vi "Go.vi"(8 "Timing Data (Go Down and Dispense)":T1(array[cluster]), 9 "Timing Data":dbl[](array[numeric]), 10 "Control In":T2={"I-O.lvclass"=refnum, "Motion.lvclass"=refnum, "Dispenser.lvclass"=refnum}, 11 "C4 Dispense in":refnum<class "Iterative Dispense.lvclass">) -> (2 "Control Out":T2, 3 "C4 Dispense Out":refnum<class "Iterative Dispense.lvclass">)   [LabVIEW 2016, in "Iterative Dispense.lvclass"]
uses:
  Iterative Dispense.lvclass
  Controller/Controllers.ctl
  Controller/I-O/I-O.lvclass
  Controller/Motion/A3200/A3200.lvclass
  Controller/Dispenser/Dispenser.lvclass
  Controller/Motion/Motion.lvclass
  Iterative Dispense.lvclass/Iterative Dispense.ctl
  Controller/Controller.lvclass
panel:
  out "deleted portion":dbl[][](array[numeric])
  out "array w/ subset deleted":dbl[][][](array[numeric])
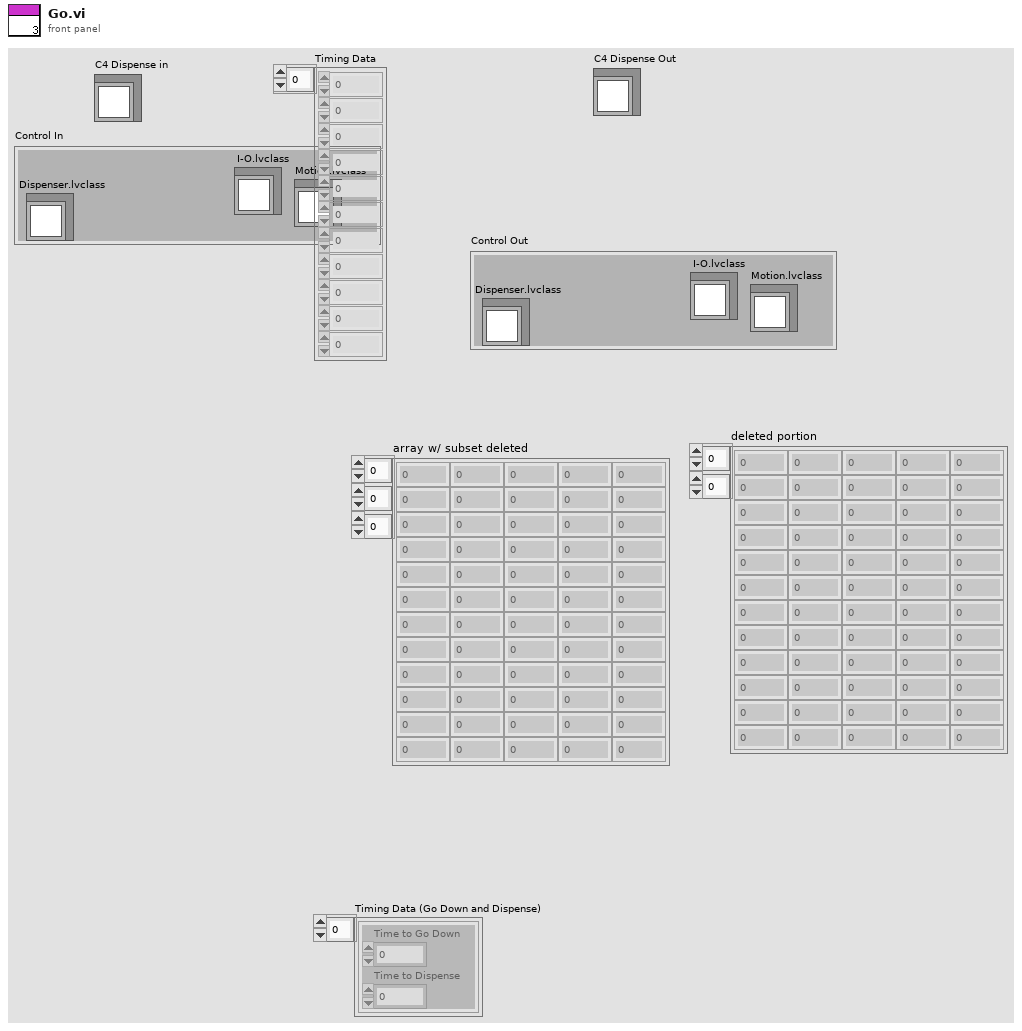
[diagram p1: front panel]
types:
  T1 = cluster{"Time to Go Down":dbl, "Time to Dispense":dbl}[]
  T2 = typedef "Controller.lvclass/Controllers.ctl" = cluster{"I-O.lvclass":refnum<class "I-O.lvclass">, "Motion.lvclass":refnum<class "Motion.lvclass">, "Dispenser.lvclass":refnum<class "Dispenser.lvclass">}
  T3 = typedef "Iterative Dispense.lvclass/Glue Step Enum.ctl" = enum16{"Baseplate to Kapton", "Kapton to Sensor"}
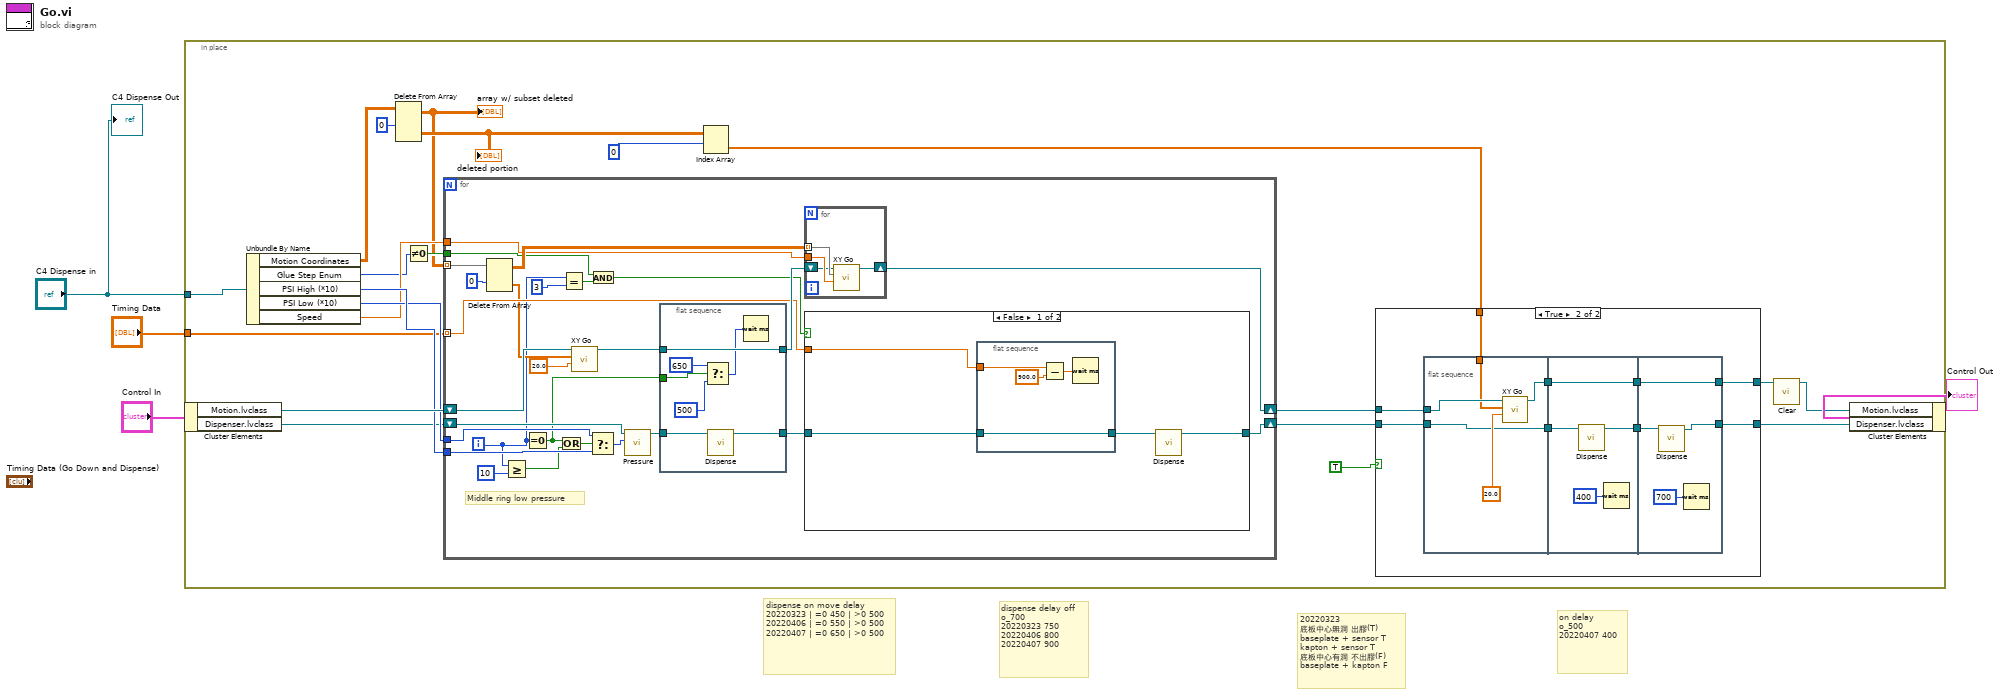
[diagram p0: block diagram]
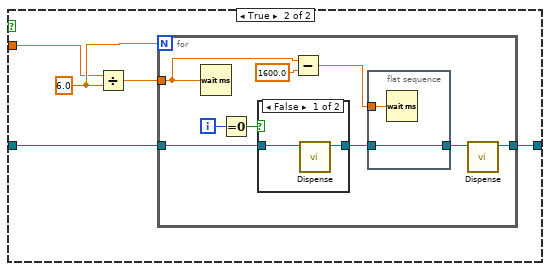
[diagram p3: hidden frame]
diagram:
  # "20220323\n底板中心無洞 出膠(T)\nbaseplate + sensor T\nkapton + sensor T\n底板中心有洞 不出膠(F)\nbaseplate + kapton F"
  # "on delay\no_500\n20220407 400"
  # "dispense delay off\no_700\n20220323 750\n20220406 800\n20220407 900"
  # "dispense on move delay\n20220323 | =0 450 | >0 500\n20220406 | =0 550 | >0 500\n20220407 | =0 650 | >0 500"
  n1 = in-place {
    in-place-border: "C4 Dispense in" -> [w12]
    in-place-border: "Timing Data" -> [w20]
    n2 = in-place-cluster #1("Control In") -> ("Motion.lvclass"=w24:refnum<class "Motion.lvclass">, "Dispenser.lvclass"=w19:refnum<class "Dispenser.lvclass">)
    n3 = Unbundle By Name(w12) -> ("Motion Coordinates"=w7:dbl[][][], "Glue Step Enum"=w18:T3, "PSI High (*10)"=w23:i32, "PSI Low (*10)"=w22:i32, "Speed"=w21:dbl)
    n4 = Delete From Array(array=w7, index (dim 0)=0 ("index (page)")) -> (deleted portion=w10:dbl[][], array with subset deleted=w6:dbl[][][])  [unwired: 3 in]
    "array w/ subset deleted" <- w6
    "deleted portion" <- w10
    n5 = Not Equal To 0?(x=w18) -> (x != 0?=w25:bool)
    n6 = for {
      tunnel: w6 -> [w72] mode=indexing
      tunnel: w25 -> [w66]
      tunnel: w21 -> [w65]
      tunnel: w20 -> [w64] mode=indexing
      tunnel: w22 -> [w63]
      tunnel: w23 -> [w62]
      shift-right: [w76] -> w16
      shift-left: w24 -> [w61]
      shift-right: [w73] -> w14
      shift-left: w19 -> [w55]
      i -> [w53]
      # "Middle ring low pressure"
      # "Executes C4 Symmetric Motion"
      n7 = Delete From Array(array=w72, index (row)=0) -> (deleted portion=w59:dbl[], array with subset deleted=w70:dbl[][])  [unwired: 2 in]
      n8 = Greater Or Equal?(x=w53, y=10) -> (x >= y?=w51:bool)
      n9 = Equal To 0?(x=w53) -> (x = 0?=w50:bool)
      n10 = Or(x=w50, y=w51) -> (x .or. y?=w54:bool)
      n11 = Equal?(x=w53, y=3) -> (x = y?=w74:bool)
      n12 = call-dynamic "XY Go.vi"("Speed"=20.0 ("speed"), "XY"=w59, "Motion in"=w61) -> ("Motion out"=w60:refnum<class "Motion.lvclass">)  [unwired: 7 in, 1 out]
      n13 = Select(t=w63, s=w54, f=w62) -> (s? t:f=w56:i32)
      n14 = And(x=w66, y=w74) -> (x .and. y?=w67:bool)
      n15 = call-dynamic "Pressure.vi"("Pressure"=w56, "Dispenser in"=w55) -> ("Dispenser out"=w57:refnum<class "Dispenser.lvclass">)  [unwired: 8 in, 1 out]
      n16 = flat-sequence {
        tunnel: w57 -> [w109]
        tunnel: w60 -> [w110]
        tunnel: [w110] -> w69
        tunnel: [w108] -> w68
        tunnel: w50 -> [w107]
        frame #0 {
          n17 = Select(t=u32 650, s=w107, f=u32 500 ("milliseconds to wait")) -> (s? t:f=w106:u32)
          n18 = call-dynamic "Dispense.vi"("Dispenser in"=w109) -> ("Dispenser out"=w108:refnum<class "Dispenser.lvclass">)  [unwired: 9 in, 1 out]
          n19 = Wait (ms)(milliseconds to wait=w106) -> ()  [unwired: 1 out]
        }
      }
      n20 = for {
        tunnel: w65 -> [w113]
        tunnel: w70 -> [w114] mode=indexing
        shift-right: [w111] -> w76
        shift-left: w69 -> [w112]
        n21 = call-dynamic "XY Go.vi"("Speed"=w113, "XY"=w114, "Motion in"=w112) -> ("Motion out"=w111:refnum<class "Motion.lvclass">)  [unwired: 7 in, 1 out]
      }
      n22 = case shown="False" w67 {
        tunnel: w64 -> [w80 w85]
        tunnel: w68 -> [w79 w88]
        tunnel: [w77 w87] -> w73
        frame False {
          n23 = flat-sequence {
            tunnel: w79 -> [w82]
            tunnel: w80 -> [w81]
            tunnel: [w82] -> w78
            frame #0 {
              n24 = Subtract(x=w81, y=900.0) -> (x-y=w84:dbl)
              n25 = Wait (ms)(milliseconds to wait=w84) -> ()  [unwired: 1 out]
            }
          }
          n26 = call-dynamic "Dispense.vi"("Dispenser in"=w78) -> ("Dispenser out"=w77:refnum<class "Dispenser.lvclass">)  [unwired: 9 in, 1 out]
        }
        frame True {
          w86 = 6.0 ("y")
          # "Leaves Space for Silver Epoxy"
          n27 = Divide(x=w85, y=w86) -> (x/y=w89:dbl)
          n28 = for {
            N: w86 -> [_]
            tunnel: w89 -> [w96]
            tunnel: w88 -> [w95]
            tunnel: [w91] -> w87
            i -> [w93]
            n29 = Wait (ms)(milliseconds to wait=w96) -> ()  [unwired: 1 out]
            n30 = Equal To 0?(x=w93) -> (x = 0?=w92:bool)
            n31 = case shown="False" w92 {
              tunnel: w95 -> [w99 w101]
              tunnel: [w100 w101] -> w94
              frame False {
                n32 = call-dynamic "Dispense.vi"("Dispenser in"=w99) -> ("Dispenser out"=w100:refnum<class "Dispenser.lvclass">)  [unwired: 9 in, 1 out]
              }
              frame True {
              }
            }
            n33 = Subtract(x=w96, y=1600.0) -> (x-y=w97:dbl)
            n34 = flat-sequence {
              tunnel: w97 -> [w103]
              tunnel: w94 -> [w102]
              tunnel: [w102] -> w90
              frame #0 {
                n35 = Wait (ms)(milliseconds to wait=w103) -> ()  [unwired: 1 out]
              }
            }
            n36 = call-dynamic "Dispense.vi"("Dispenser in"=w90) -> ("Dispenser out"=w91:refnum<class "Dispenser.lvclass">)  [unwired: 9 in, 1 out]
          }
        }
      }
    }
    n37 = Index Array(array=w10, index (row)=0) -> (element=w8:dbl[])  [unwired: 1 in]
    n38 = case shown="True" TRUE {
      tunnel: w16 -> [w27 w36]
      tunnel: [w27 w35] -> w15
      tunnel: w14 -> [w26 w34]
      tunnel: [w26 w33] -> w13
      tunnel: w8 -> [_ w32]
      frame False {
      }
      frame True {
        n39 = flat-sequence {
          tunnel: w36 -> [w40]
          tunnel: w34 -> [w38]
          tunnel: [w39] -> w31
          tunnel: [w38] -> w30
          tunnel: w32 -> [w37]
          tunnel: w31 -> [w45]
          tunnel: w30 -> [w44]
          tunnel: [w45] -> w29
          tunnel: [w42] -> w28
          tunnel: [w49] -> w35
          tunnel: w29 -> [w49]
          tunnel: w28 -> [w47]
          tunnel: [w46] -> w33
          frame #0 {
            n40 = call-dynamic "XY Go.vi"("Speed"=20.0 ("speed"), "XY"=w37, "Motion in"=w40) -> ("Motion out"=w39:refnum<class "Motion.lvclass">)  [unwired: 7 in, 1 out]
          }
          frame #1 {
            n41 = call-dynamic "Dispense.vi"("Dispenser in"=w44) -> ("Dispenser out"=w42:refnum<class "Dispenser.lvclass">)  [unwired: 9 in, 1 out]
            n42 = Wait (ms)(milliseconds to wait=u32 400) -> ()  [unwired: 1 out]
          }
          frame #2 {
            n43 = call-dynamic "Dispense.vi"("Dispenser in"=w47) -> ("Dispenser out"=w46:refnum<class "Dispenser.lvclass">)  [unwired: 9 in, 1 out]
            n44 = Wait (ms)(milliseconds to wait=u32 700) -> ()  [unwired: 1 out]
          }
        }
      }
    }
    n45 = call "Clear.vi"("Motion in"=w15) -> ("Motion out"=w17:refnum<class "Motion.lvclass">)  [unwired: 9 in, 1 out]
    n46 = in-place-cluster #1("Motion.lvclass"=w17, "Dispenser.lvclass"=w13) -> (→"Control Out":T2)
  }
  "C4 Dispense Out" <- "C4 Dispense in"
